vi "滤波器消噪.vi"(0 "滤波器选择":u16(ring) items=["切比雪夫", "巴特沃斯"], 1 "滤波器类型":i32(ring) items=["低通", "高通", "带通", "带阻"], 2 "高截止频率":dbl=8000.0 format="%.2f", 3 "低截止频率":dbl=60.0 format="%.2f", 4 "阶数":dbl=2.0 format="%.2f") -> (5 "?":cluster{i32, dbl, dbl[]}(graph), 6 "?":dbl[](graph), 7 "?":cluster{i32, dbl, dbl[]}(graph), 8 "Time Waveform":dbl[](graph))   [LabVIEW 2013]
uses:
  <vilib>/sound/lvsound.llb/Sound Format.ctl
  <vilib>/Analysis/2dsp.llb/Real FFT.vi
  <vilib>/Analysis/3filter.llb/Chebyshev Filter (DBL).vi
  <vilib>/Analysis/3filter.llb/Butterworth Filter (DBL).vi
  <vilib>/Analysis/NI_AALPro.lvlib
  <vilib>/Analysis/NI_AALBase.lvlib
panel:
  in  "Buffer Size":u32=8192
  in  "stop":bool
  # "语音信号实时采集、消噪"
  # "原 始 语 音 信 号"
  # "语 音 信 号 的 频 谱"
  # "滤 波 器 消 噪"
  # "滤 波 器 选 择 与 调 控"
  # "消噪后语音信号频谱图"
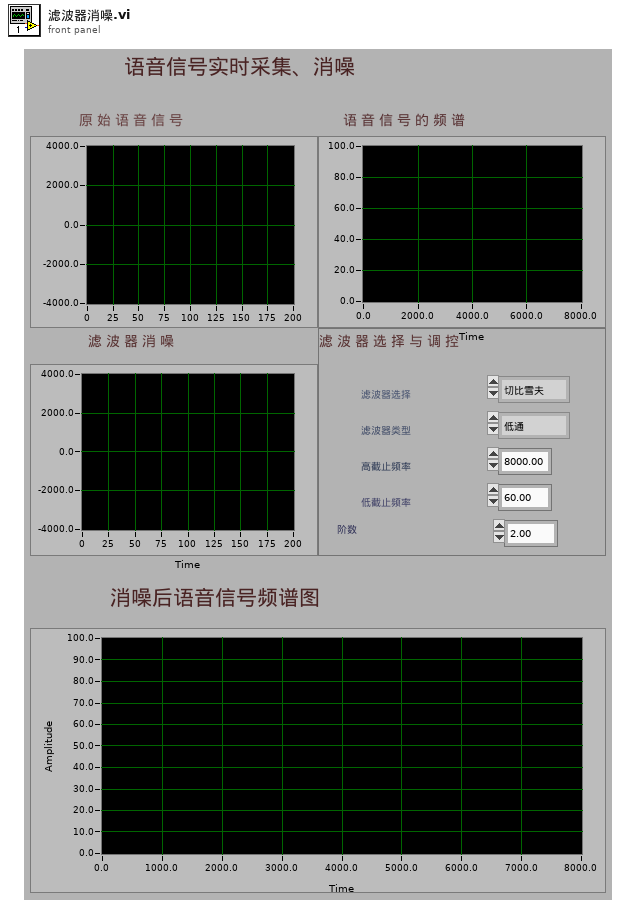
[diagram p1: front panel]
types:
  T1 = typedef "Sound Format.ctl" = cluster{"sound quality":enum16{"mono", "stereo"}, "rate":enum16{"11025", "22050", "44100", "8000"}, "bits per sample":enum16{"8 bit", "16 bit"}}
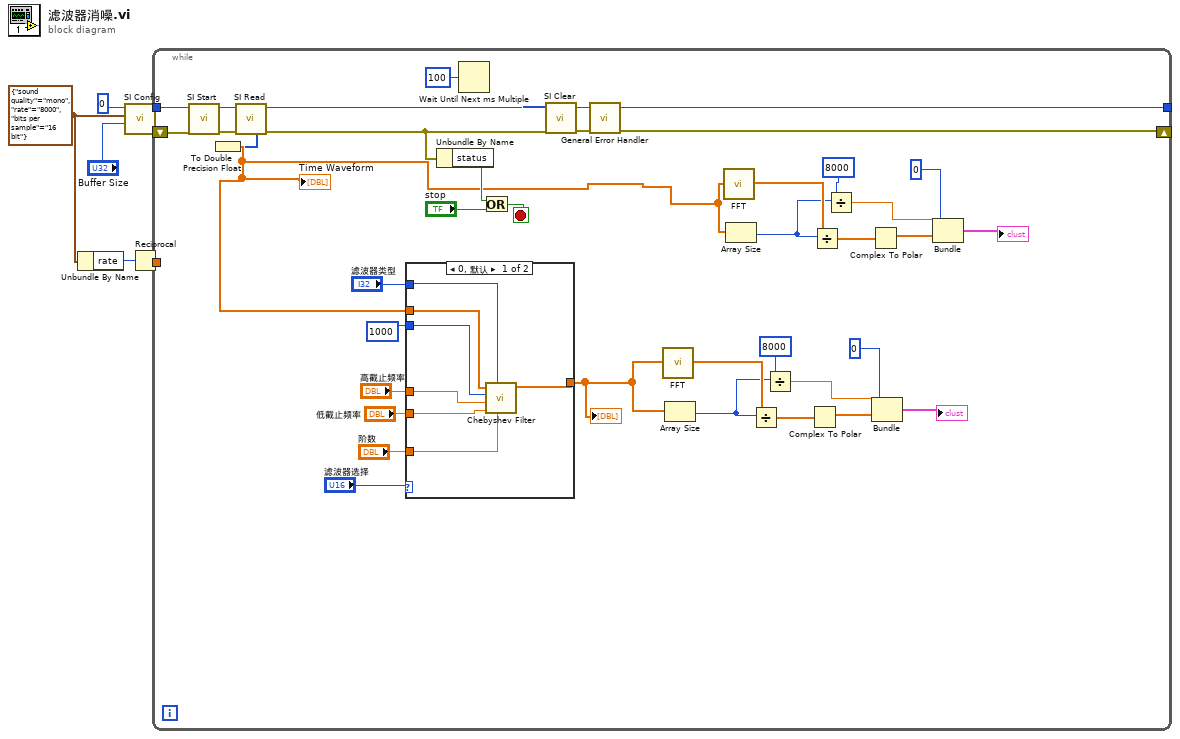
[diagram p0: block diagram]
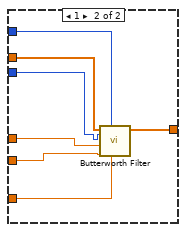
[diagram p2: hidden frame]
diagram:
  w2 = T1 {"sound quality"=enum."mono", "rate"=enum."8000", "bits per sample"=enum."16 bit"} ("sound format")
  n1 = Unbundle By Name(w2) -> ("rate"=w1:enum16{"11025", "22050", "44100", "8000"})
  n2 = call <vilib>:"SI Config.vi"("buffer size (8192 in bytes)"="Buffer Size", "sound format"=w2, "device (0)"=u32 0 ("device")) -> ("error out"=w5:errorcluster, "task ID out"=w9:u32)  [unwired: 7 in]
  n3 = Reciprocal(x=w1) -> (1/x=w7:dbl)
  n4 = while {
    shift-left: w5 -> [w41]
    shift-right: [w40] -> w4
    tunnel: w9 -> [w43]
    tunnel: [w42] -> w8
    tunnel: w7 -> [_]
    stop <- w36 stop-if-true
    n5 = call <vilib>:"SI Start.vi"("error in (no error)"=w41, "task ID in"=w43) -> ("error out"=w44:errorcluster, "task ID out"=w45:u32)  [unwired: 8 in]
    n6 = call <vilib>:"SI Read.vi"("error in (no error)"=w44, "task ID in"=w45) -> ("error out"=w40:errorcluster, "task ID out"=w42:u32, "mono 16-bit"=w11:i16[])  [unwired: 4 in, 3 out]
    n7 = To Double Precision Float(number=w11) -> (double precision float=w21:dbl[])
    "Time Waveform" <- w21
    n8 = case shown="0, 默认" "滤波器选择" {
      tunnel: "滤波器类型" -> [w47 w59]
      tunnel: "高截止频率" -> [w52 w56]
      tunnel: "低截止频率" -> [w51 w55]
      tunnel: "阶数" -> [w50 w54]
      tunnel: 1000 -> [w49 w57]
      tunnel: w21 -> [w48 w58]
      tunnel: [w46 w53] -> w12
      frame 0, Default {
        n9 = call-poly <vilib>:"Chebyshev Filter.vi"("ripple(dB)"=w50, "filter type"=w47, "low cutoff freq: fl"=w51, "high cutoff freq: fh"=w52, "sampling freq: fs"=w49, "X"=w48) -> ("Filtered X"=w46:dbl[])  [unwired: 4 in, 1 out]
      }
      frame 1 {
        n10 = call-poly <vilib>:"Butterworth Filter.vi"("order"=w54, "filter type"=w59, "low cutoff freq: fl"=w55, "high cutoff freq: fh"=w56, "sampling freq: fs"=w57, "X"=w58) -> ("Filtered X"=w53:dbl[])  [unwired: 2 in, 1 out]
      }
    }
    "?" <- w12
    n11 = Unbundle By Name(w40) -> ("status"=w38:bool)
    n12 = Wait Until Next ms Multiple(millisecond multiple=u32 100) -> ()  [unwired: 1 out]
    n13 = Or(x=w38, y="stop") -> (x .or. y?=w36:bool)
    n14 = call-poly <vilib>:"FFT.vi"("X"=w12) -> ("FFT {X}"=w20:cdb[])  [unwired: 9 in, 1 out]
    n15 = Array Size(array=w12) -> (size(s)=w13:i32)
    n16 = call-poly <vilib>:"FFT.vi"("X"=w21) -> ("FFT {X}"=w35:cdb[])  [unwired: 9 in, 1 out]
    n17 = Array Size(array=w21) -> (size(s)=w28:i32)
    n18 = Divide(x=w20, y=w13) -> (x/y=w18:cdb[])
    n19 = Divide(x=8000, y=w13) -> (x/y=w16:dbl)
    n20 = Complex To Polar(r * e^(i*theta)=w18) -> (r=w17:dbl[])  [unwired: 1 out]
    n21 = Divide(x=w35, y=w28) -> (x/y=w33:cdb[])
    n22 = Divide(x=8000, y=w28) -> (x/y=w31:dbl)
    n23 = Complex To Polar(r * e^(i*theta)=w33) -> (r=w32:dbl[])  [unwired: 1 out]
    n24 = Bundle(0, w16, w17) -> (→"?":cluster{i32, dbl, dbl[]})  [unwired: 1 in]
    n25 = Bundle(0, w31, w32) -> (→"?":cluster{i32, dbl, dbl[]})  [unwired: 1 in]
  }
  n26 = call <vilib>:"SI Clear.vi"("error in (no error)"=w4, "task ID in"=w8) -> ("error out"=w3:errorcluster)  [unwired: 9 in]
  n27 = call <vilib>:"General Error Handler.vi"("error in (no error)"=w3) -> ()  [unwired: 10 in, 5 out]
